vi "Check Status No Objects - Function Generator.vi"(8 "error in (no error)":errorcluster, 10 "VISA Resource Name":refnum<visa-resource-name>="USB0::0x0699::0x0345::C010595::INSTR", 11 "Input Cluster":T3={"Ch2"={"General Settings"={" Frequency"=0.0, " Phase"=0.0, " Run Mode"=0, " Waveform Shape"=0, "Output on?"=FALSE}, "Voltage Settings"={"Amplitude"=0.0, "Offset"=0.0}, "Ramp Settings"={"Ramp Symmetry (%)"=50.0}, "Pulse Settings"={"Leading Edge Time "=5e-09, "Trailing Edge Time"=5e-09, "Duty Cycle (%)"=50.0}, "Sweep Mode Settings"={"Start Freq. "=0.0, "Stop Freq.  "=0.0, "Sweep spacing"=0, "Sweep time"=0.0, "Hold time"=0.0, "Return time"=0.0}, "Burst Mode Settings"={"Burst Mode "=1, "Burst Count"=5}, "AM Settings"={"AM Source "=0, "Modulation Waveform "=0, "Modulation Frequency "=1000.0, "Modulation Depth "=0.0}, "FM Settings"={"FM Source "=0, "Modulation Waveform "=0, "Modulation Frequency"=100.0, "Peak Deviation "=100.0}}, "Ch1"={"General Settings"={" Frequency"=0.0, " Phase"=0.0, " Run Mode"=0, " Waveform Shape"=0, "Output on?"=FALSE}, "Voltage Settings"={"Amplitude"=0.0, "Offset"=0.0}, "Ramp Settings"={"Ramp Symmetry (%)"=50.0}, "Pulse Settings"={"Leading Edge Time "=5e-09, "Trailing Edge Time"=5e-09, "Duty Cycle (%)"=50.0}, "Sweep Mode Settings"={"Start Freq. "=0.0, "Stop Freq.  "=0.0, "Sweep spacing"=0, "Sweep time"=0.0, "Hold time"=0.0, "Return time"=0.0}, "Burst Mode Settings"={"Burst Mode "=1, "Burst Count"=5}, "AM Settings"={"AM Source "=0, "Modulation Waveform "=0, "Modulation Frequency "=1000.0, "Modulation Depth "=0.0}, "FM Settings"={"FM Source "=0, "Modulation Waveform "=0, "Modulation Frequency"=100.0, "Peak Deviation "=100.0}}} {"Ch1"."General Settings"."Waveform Shape" items=["Sinusoid", "Square", "Pulse", "Ramp", "PRNoise", "DC", "SINC", "Gaussian", "Lorentz", "ERise", "EDecay", "Haversine", "User 1", "User 2", "User 3", "User 4", "EMemory", "EFile"]; "Ch1"."General Settings"."Run Mode" items=["Continuous", "AM", "FM", "PM", "FSK", "PWM", "Sweep", "Burst"]; "Ch1"."FM Settings"."Modulation Waveform" items=["Sine", "Square", "Triangle", "Ramp", "Down Ramp", "Noise", "User 1", "User 2", "User 3", "User 4", "EMEMory", "EFILe"]; "Ch1"."FM Settings"."FM Source" items=["Internal", "External"]; "Ch1"."AM Settings"."Modulation Waveform" items=["Sine", "Square", "Triangle", "Ramp", "Down Ramp", "Noise"]; "Ch1"."AM Settings"."AM Source" items=["Internal", "External"]; "Ch1"."Burst Mode Settings"."Burst Mode" items=["Triggered", "Gated"]; "Ch1"."Sweep Mode Settings"."Sweep spacing" items=["linear", "log"]; "Ch1"."Pulse Settings"."Trailing Edge Time" format="%#.6g"; "Ch1"."Pulse Settings"."Leading Edge Time" format="%#.6g"; "Ch1"."Ramp Settings"."Ramp Symmetry (%)" min=0.0 max=100.0 step=1.0 format="%.2f"; "Ch2"."General Settings"."Waveform Shape" items=["Sinusoid", "Square", "Pulse", "Ramp", "PRNoise", "DC", "SINC", "Gaussian", "Lorentz", "ERise", "EDecay", "Haversine", "User 1", "User 2", "User 3", "User 4", "EMemory", "EFile"]; "Ch2"."General Settings"."Run Mode" items=["Continuous", "AM", "FM", "PM", "FSK", "PWM", "Sweep", "Burst"]; "Ch2"."FM Settings"."Modulation Waveform" items=["Sine", "Square", "Triangle", "Ramp", "Down Ramp", "Noise", "User 1", "User 2", "User 3", "User 4", "EMEMory", "EFILe"]; "Ch2"."FM Settings"."FM Source" items=["Internal", "External"]; "Ch2"."AM Settings"."Modulation Waveform" items=["Sine", "Square", "Triangle", "Ramp", "Down Ramp", "Noise"]; "Ch2"."AM Settings"."AM Source" items=["Internal", "External"]; "Ch2"."Burst Mode Settings"."Burst Mode" items=["Triggered", "Gated"]; "Ch2"."Sweep Mode Settings"."Sweep spacing" items=["linear", "log"]; "Ch2"."Pulse Settings"."Trailing Edge Time" format="%#.6g"; "Ch2"."Pulse Settings"."Leading Edge Time" format="%#.6g"; "Ch2"."Ramp Settings"."Ramp Symmetry (%)" min=0.0 max=100.0 step=1.0 format="%.2f"}) -> (0 "error out":errorcluster, 1 "Status":string, 2 "Ready?":bool, 3 "Output Cluster":T3={"Ch2"={"General Settings"={" Frequency"=0.0, " Phase"=0.0, " Run Mode"=0, " Waveform Shape"=0, "Output on?"=FALSE}, "Voltage Settings"={"Amplitude"=0.0, "Offset"=0.0}, "Ramp Settings"={"Ramp Symmetry (%)"=50.0}, "Pulse Settings"={"Leading Edge Time "=5e-09, "Trailing Edge Time"=5e-09, "Duty Cycle (%)"=50.0}, "Sweep Mode Settings"={"Start Freq. "=0.0, "Stop Freq.  "=0.0, "Sweep spacing"=0, "Sweep time"=0.0, "Hold time"=0.0, "Return time"=0.0}, "Burst Mode Settings"={"Burst Mode "=1, "Burst Count"=5}, "AM Settings"={"AM Source "=0, "Modulation Waveform "=0, "Modulation Frequency "=1000.0, "Modulation Depth "=0.0}, "FM Settings"={"FM Source "=0, "Modulation Waveform "=0, "Modulation Frequency"=100.0, "Peak Deviation "=100.0}}, "Ch1"={"General Settings"={" Frequency"=0.0, " Phase"=0.0, " Run Mode"=0, " Waveform Shape"=0, "Output on?"=FALSE}, "Voltage Settings"={"Amplitude"=0.0, "Offset"=0.0}, "Ramp Settings"={"Ramp Symmetry (%)"=50.0}, "Pulse Settings"={"Leading Edge Time "=5e-09, "Trailing Edge Time"=5e-09, "Duty Cycle (%)"=50.0}, "Sweep Mode Settings"={"Start Freq. "=0.0, "Stop Freq.  "=0.0, "Sweep spacing"=0, "Sweep time"=0.0, "Hold time"=0.0, "Return time"=0.0}, "Burst Mode Settings"={"Burst Mode "=1, "Burst Count"=5}, "AM Settings"={"AM Source "=0, "Modulation Waveform "=0, "Modulation Frequency "=1000.0, "Modulation Depth "=0.0}, "FM Settings"={"FM Source "=0, "Modulation Waveform "=0, "Modulation Frequency"=100.0, "Peak Deviation "=100.0}}} {"Ch1"."General Settings"."Waveform Shape" items=["Sinusoid", "Square", "Pulse", "Ramp", "PRNoise", "DC", "SINC", "Gaussian", "Lorentz", "ERise", "EDecay", "Haversine", "User 1", "User 2", "User 3", "User 4", "EMemory", "EFile"]; "Ch1"."General Settings"."Run Mode" items=["Continuous", "AM", "FM", "PM", "FSK", "PWM", "Sweep", "Burst"]; "Ch1"."FM Settings"."Modulation Waveform" items=["Sine", "Square", "Triangle", "Ramp", "Down Ramp", "Noise", "User 1", "User 2", "User 3", "User 4", "EMEMory", "EFILe"]; "Ch1"."FM Settings"."FM Source" items=["Internal", "External"]; "Ch1"."AM Settings"."Modulation Waveform" items=["Sine", "Square", "Triangle", "Ramp", "Down Ramp", "Noise"]; "Ch1"."AM Settings"."AM Source" items=["Internal", "External"]; "Ch1"."Burst Mode Settings"."Burst Mode" items=["Triggered", "Gated"]; "Ch1"."Sweep Mode Settings"."Sweep spacing" items=["linear", "log"]; "Ch1"."Pulse Settings"."Trailing Edge Time" format="%#.6g"; "Ch1"."Pulse Settings"."Leading Edge Time" format="%#.6g"; "Ch1"."Ramp Settings"."Ramp Symmetry (%)" min=0.0 max=100.0 step=1.0 format="%.2f"; "Ch2"."General Settings"."Waveform Shape" items=["Sinusoid", "Square", "Pulse", "Ramp", "PRNoise", "DC", "SINC", "Gaussian", "Lorentz", "ERise", "EDecay", "Haversine", "User 1", "User 2", "User 3", "User 4", "EMemory", "EFile"]; "Ch2"."General Settings"."Run Mode" items=["Continuous", "AM", "FM", "PM", "FSK", "PWM", "Sweep", "Burst"]; "Ch2"."FM Settings"."Modulation Waveform" items=["Sine", "Square", "Triangle", "Ramp", "Down Ramp", "Noise", "User 1", "User 2", "User 3", "User 4", "EMEMory", "EFILe"]; "Ch2"."FM Settings"."FM Source" items=["Internal", "External"]; "Ch2"."AM Settings"."Modulation Waveform" items=["Sine", "Square", "Triangle", "Ramp", "Down Ramp", "Noise"]; "Ch2"."AM Settings"."AM Source" items=["Internal", "External"]; "Ch2"."Burst Mode Settings"."Burst Mode" items=["Triggered", "Gated"]; "Ch2"."Sweep Mode Settings"."Sweep spacing" items=["linear", "log"]; "Ch2"."Pulse Settings"."Trailing Edge Time" format="%#.6g"; "Ch2"."Pulse Settings"."Leading Edge Time" format="%#.6g"; "Ch2"."Ramp Settings"."Ramp Symmetry (%)" min=0.0 max=100.0 step=1.0 format="%.2f"})   [LabVIEW 2012]
doc: "Checks if the instrument is powered on and updates its member data with the instrument's current status."
uses:
  Tektronix AFG 3000 Series/controls.llb/Waveform Shape.ctl
  Tektronix AFG 3000 Series/controls.llb/Sweep Spacing.ctl
  Tektronix AFG 3000 Series/controls.llb/Sweep Time Parameter.ctl
  Tektronix AFG 3000 Series/controls.llb/Sweep Frequency.ctl
  Tektronix AFG 3000 Series/controls.llb/Voltage.ctl
  Tektronix AFG 3000 Series/Tektronix AFG 3000 Series.lvlib
panel:
  in  "Channel Settings":T4={"General Settings"={" Frequency"=0.0, " Phase"=0.0, " Run Mode"=0, " Waveform Shape"=0, "Output on?"=FALSE}, "Voltage Settings"={"Amplitude"=0.0, "Offset"=0.0}, "Ramp Settings"={"Ramp Symmetry (%)"=50.0}, "Pulse Settings"={"Leading Edge Time "=5e-09, "Trailing Edge Time"=5e-09, "Duty Cycle (%)"=50.0}, "Sweep Mode Settings"={"Start Freq. "=0.0, "Stop Freq.  "=0.0, "Sweep spacing"=0, "Sweep time"=0.0, "Hold time"=0.0, "Return time"=0.0}, "Burst Mode Settings"={"Burst Mode "=1, "Burst Count"=5}, "AM Settings"={"AM Source "=0, "Modulation Waveform "=0, "Modulation Frequency "=1000.0, "Modulation Depth "=0.0}, "FM Settings"={"FM Source "=0, "Modulation Waveform "=0, "Modulation Frequency"=100.0, "Peak Deviation "=100.0}} {"General Settings"."Waveform Shape" items=["Sinusoid", "Square", "Pulse", "Ramp", "PRNoise", "DC", "SINC", "Gaussian", "Lorentz", "ERise", "EDecay", "Haversine", "User 1", "User 2", "User 3", "User 4", "EMemory", "EFile"]; "General Settings"."Run Mode" items=["Continuous", "AM", "FM", "PM", "FSK", "PWM", "Sweep", "Burst"]; "FM Settings"."Modulation Waveform" items=["Sine", "Square", "Triangle", "Ramp", "Down Ramp", "Noise", "User 1", "User 2", "User 3", "User 4", "EMEMory", "EFILe"]; "FM Settings"."FM Source" items=["Internal", "External"]; "AM Settings"."Modulation Waveform" items=["Sine", "Square", "Triangle", "Ramp", "Down Ramp", "Noise"]; "AM Settings"."AM Source" items=["Internal", "External"]; "Burst Mode Settings"."Burst Mode" items=["Triggered", "Gated"]; "Sweep Mode Settings"."Sweep spacing" items=["linear", "log"]; "Pulse Settings"."Trailing Edge Time" format="%#.6g"; "Pulse Settings"."Leading Edge Time" format="%#.6g"; "Ramp Settings"."Ramp Symmetry (%)" min=0.0 max=100.0 step=1.0 format="%.2f"}
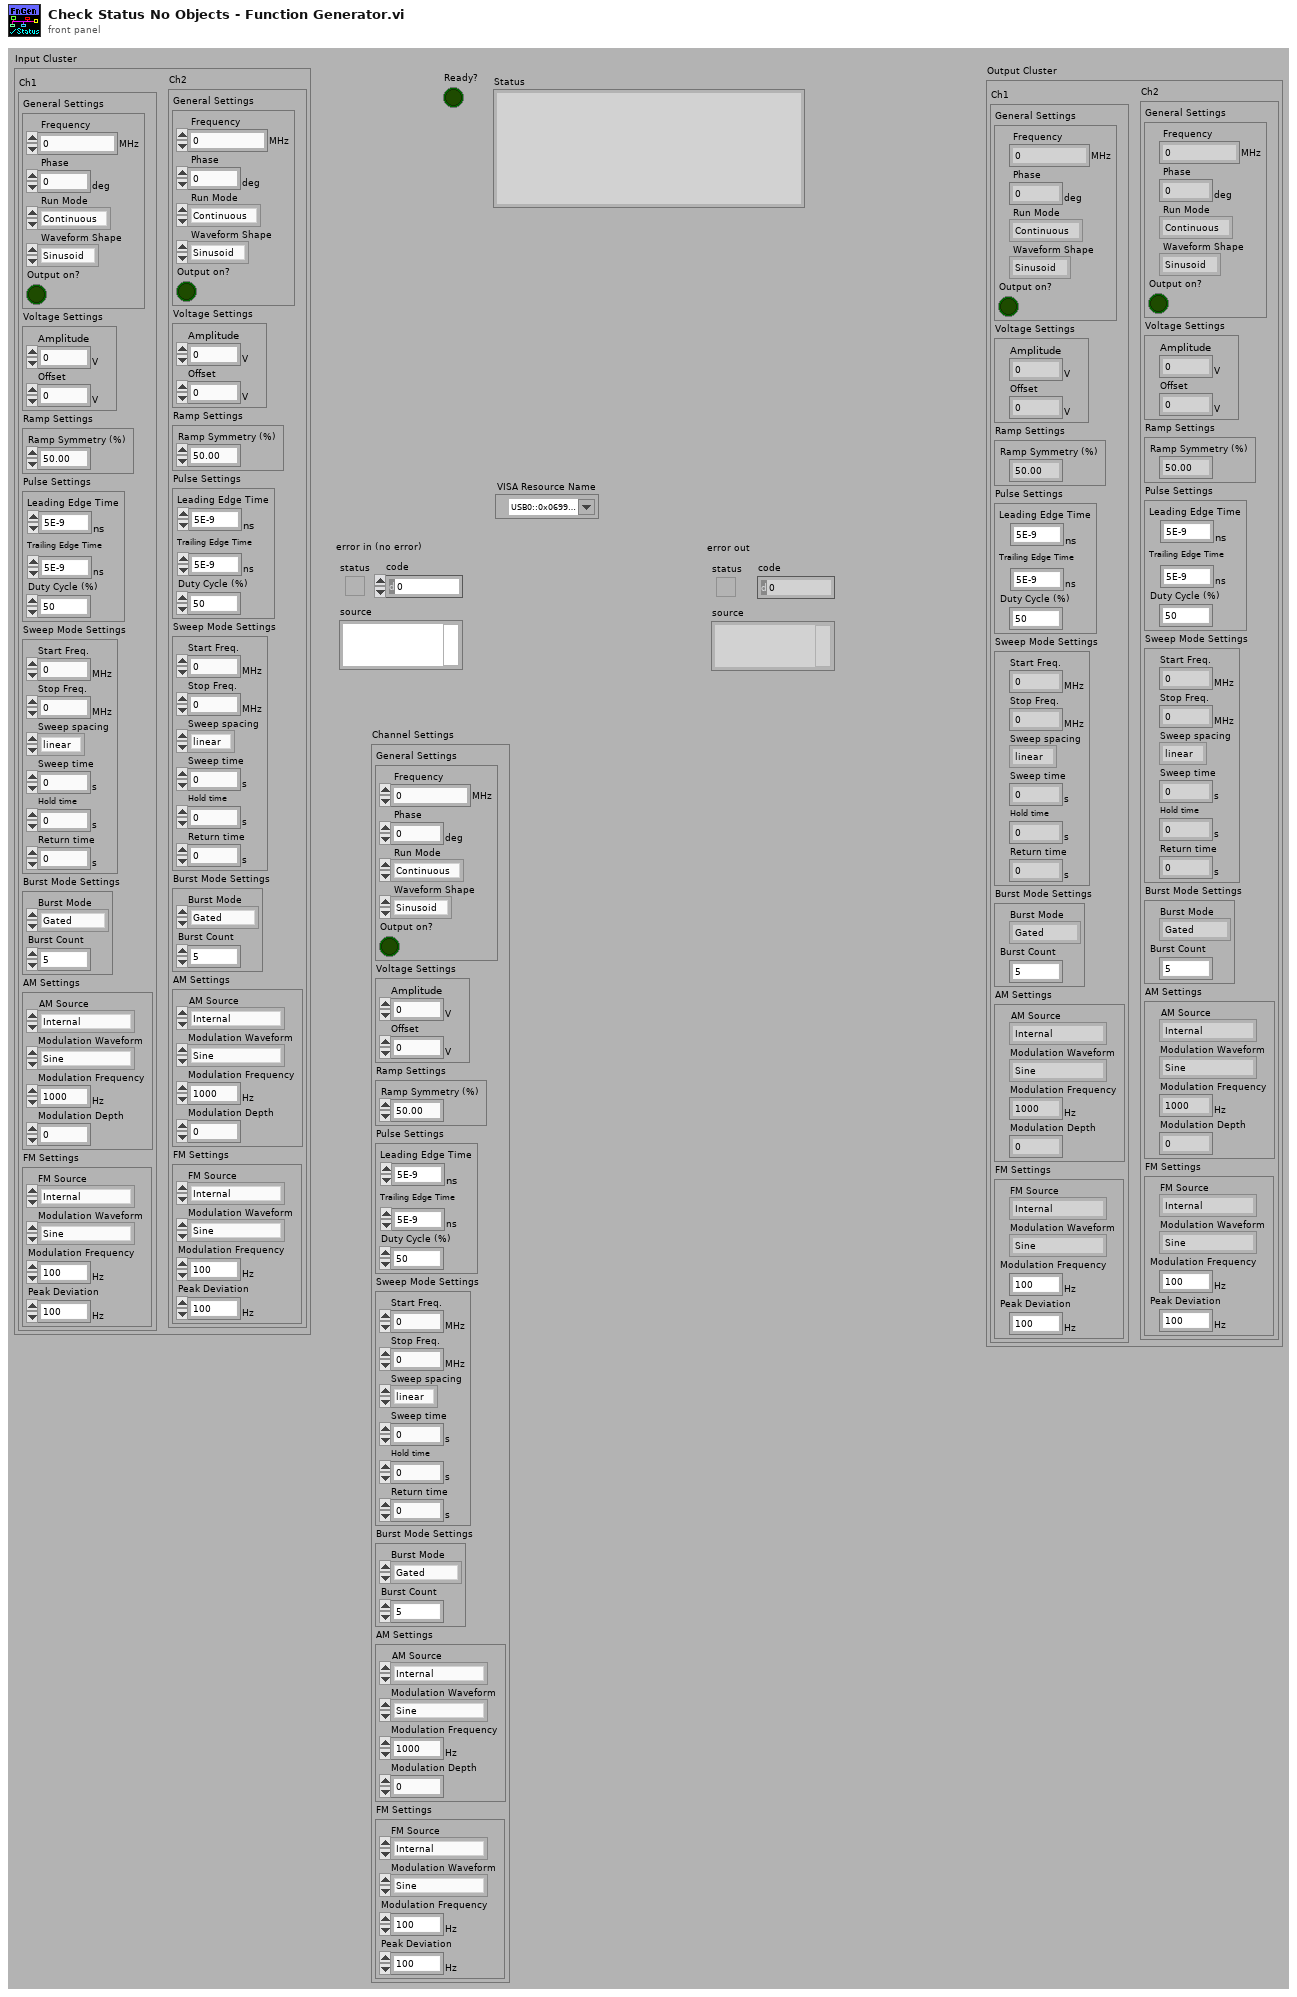
[diagram p1: front panel]
types:
  T1 = typedef "Waveform Shape.ctl" = u16
  T2 = typedef "Sweep Spacing.ctl" = u16
  T3 = cluster{"Ch2":cluster{"General Settings":cluster{" Frequency":dbl[unit], " Phase":dbl[unit], " Run Mode":u16, " Waveform Shape":T1, "Output on?":bool}, "Voltage Settings":cluster{"Amplitude":dbl[unit], "Offset":dbl[unit]}, "Ramp Settings":cluster{"Ramp Symmetry (%)":dbl}, "Pulse Settings":cluster{"Leading Edge Time ":dbl[unit], "Trailing Edge Time":dbl[unit], "Duty Cycle (%)":dbl}, "Sweep Mode Settings":cluster{"Start Freq. ":dbl[unit], "Stop Freq.  ":dbl[unit], "Sweep spacing":T2, "Sweep time":dbl[unit], "Hold time":dbl[unit], "Return time":dbl[unit]}, "Burst Mode Settings":cluster{"Burst Mode ":u16, "Burst Count":i32}, "AM Settings":cluster{"AM Source ":u16, "Modulation Waveform ":u16, "Modulation Frequency ":dbl[unit], "Modulation Depth ":dbl}, "FM Settings":cluster{"FM Source ":u16, "Modulation Waveform ":u16, "Modulation Frequency":dbl[unit], "Peak Deviation ":dbl[unit]}}, "Ch1":cluster{"General Settings":cluster{" Frequency":dbl[unit], " Phase":dbl[unit], " Run Mode":u16, " Waveform Shape":T1, "Output on?":bool}, "Voltage Settings":cluster{"Amplitude":dbl[unit], "Offset":dbl[unit]}, "Ramp Settings":cluster{"Ramp Symmetry (%)":dbl}, "Pulse Settings":cluster{"Leading Edge Time ":dbl[unit], "Trailing Edge Time":dbl[unit], "Duty Cycle (%)":dbl}, "Sweep Mode Settings":cluster{"Start Freq. ":dbl[unit], "Stop Freq.  ":dbl[unit], "Sweep spacing":T2, "Sweep time":dbl[unit], "Hold time":dbl[unit], "Return time":dbl[unit]}, "Burst Mode Settings":cluster{"Burst Mode ":u16, "Burst Count":i32}, "AM Settings":cluster{"AM Source ":u16, "Modulation Waveform ":u16, "Modulation Frequency ":dbl[unit], "Modulation Depth ":dbl}, "FM Settings":cluster{"FM Source ":u16, "Modulation Waveform ":u16, "Modulation Frequency":dbl[unit], "Peak Deviation ":dbl[unit]}}}
  T4 = cluster{"General Settings":cluster{" Frequency":dbl[unit], " Phase":dbl[unit], " Run Mode":u16, " Waveform Shape":T1, "Output on?":bool}, "Voltage Settings":cluster{"Amplitude":dbl[unit], "Offset":dbl[unit]}, "Ramp Settings":cluster{"Ramp Symmetry (%)":dbl}, "Pulse Settings":cluster{"Leading Edge Time ":dbl[unit], "Trailing Edge Time":dbl[unit], "Duty Cycle (%)":dbl}, "Sweep Mode Settings":cluster{"Start Freq. ":dbl[unit], "Stop Freq.  ":dbl[unit], "Sweep spacing":T2, "Sweep time":dbl[unit], "Hold time":dbl[unit], "Return time":dbl[unit]}, "Burst Mode Settings":cluster{"Burst Mode ":u16, "Burst Count":i32}, "AM Settings":cluster{"AM Source ":u16, "Modulation Waveform ":u16, "Modulation Frequency ":dbl[unit], "Modulation Depth ":dbl}, "FM Settings":cluster{"FM Source ":u16, "Modulation Waveform ":u16, "Modulation Frequency":dbl[unit], "Peak Deviation ":dbl[unit]}}
  T5 = typedef "Voltage.ctl" = enum16{"amplitude", "offset", "high", "low", "high limit", "low limit"}
  T6 = typedef "Sweep Frequency.ctl" = enum16{"center", "span", "start", "stop"}
  T7 = typedef "Sweep Time Parameter.ctl" = enum16{"sweep time", "hold time", "return time"}
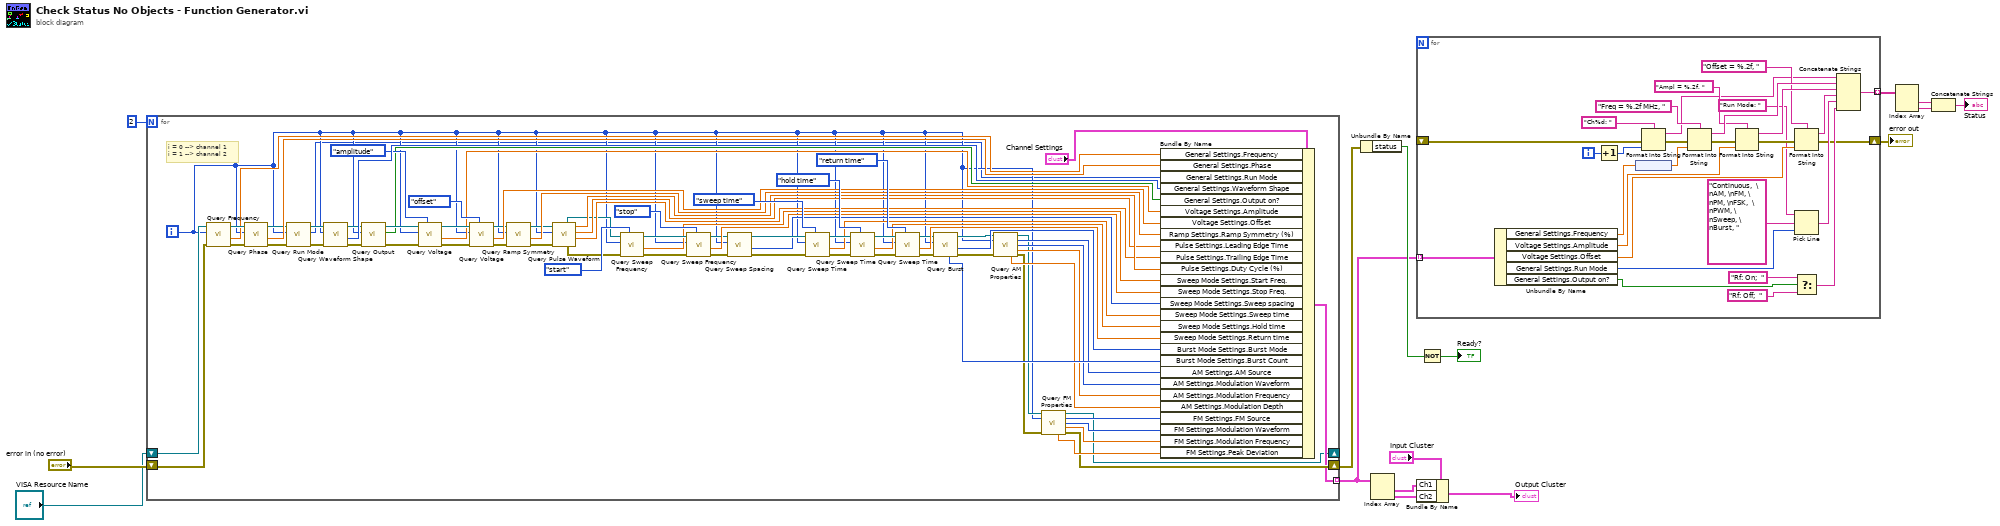
[diagram p0: block diagram]
diagram:
  n1 = for {
    N: 2 -> [_]
    shift-right: [w33] -> w14
    shift-left: "error in (no error)" -> [w82]
    tunnel: [w32] -> w13 mode=indexing
    shift-right: [w31] -> _
    shift-left: "VISA Resource Name" -> [w30]
    i -> [w19]
    # "i = 0 --> channel 1\ni = 1 --> channel 2"
    n2 = call "Query Frequency.vi"("error in (no error)"=w82, "Channel (0: Channel 1)"=w19, "VISA resource name"=w30) -> ("error out"=w81:errorcluster, "frequency"=w80:dbl[unit], "VISA resource name out"=w88:refnum<visa-resource-name>)  [unwired: 6 out]
    n3 = call "Query Phase.vi"("error in (no error)"=w81, "Channel (0: Channel 1)"=w19, "VISA resource name"=w88) -> ("error out"=w21:errorcluster, "phase"=w79:dbl[unit], "VISA resource name out"=w23:refnum<visa-resource-name>)  [unwired: 6 out]
    n4 = call "Query Run Mode.vi"("error in (no error)"=w21, "Channel (0: Channel 1)"=w19, "VISA resource name"=w23) -> ("error out"=w20:errorcluster, "Run Mode"=w18:u16, "VISA resource name out"=w22:refnum<visa-resource-name>)  [unwired: 6 out]
    n5 = call "Query Waveform Shape.vi"("error in (no error)"=w20, "Channel (0: Channel 1)"=w19, "VISA resource name"=w22) -> ("error out"=w26:errorcluster, "Waveform Shape"=w78:T1, "VISA resource name out"=w28:refnum<visa-resource-name>)  [unwired: 6 out]
    n6 = call "Query Output.vi"("error in (no error)"=w26, "Channel (0: Channel 1)"=w19, "VISA resource name"=w28) -> ("error out"=w25:errorcluster, "Output Enabled?"=w24:bool, "VISA resource name out"=w27:refnum<visa-resource-name>)  [unwired: 6 out]
    n7 = call "Query Voltage.vi"("Voltage Param (amplitude)"=Voltage."amplitude", "error in (no error)"=w25, "Channel (0: Channel 1)"=w19, "VISA resource name"=w27) -> ("error out"=w45:errorcluster, "voltage"=w29:dbl[unit], "VISA resource name out"=w75:refnum<visa-resource-name>)  [unwired: 5 out]
    n8 = call "Query Voltage.vi"("Voltage Param (amplitude)"=Voltage."offset", "error in (no error)"=w45, "Channel (0: Channel 1)"=w19, "VISA resource name"=w75) -> ("error out"=w44:errorcluster, "voltage"=w74:dbl[unit], "VISA resource name out"=w73:refnum<visa-resource-name>)  [unwired: 5 out]
    n9 = call "Query Ramp Symmetry.vi"("error in (no error)"=w44, "Channel (0: Channel 1)"=w19, "VISA resource name"=w73) -> ("error out"=w43:errorcluster, "Symmetry (%)"=w72:dbl, "VISA resource name out"=w71:refnum<visa-resource-name>)  [unwired: 6 out]
    n10 = call "Query Pulse Waveform.vi"("error in (no error)"=w43, "Channel (0: Channel 1)"=w19, "VISA resource name"=w71) -> ("Trailing"=w68:dbl[unit], "Leading"=w69:dbl[unit], "Duty Cycle"=w70:dbl, "error out"=w42:errorcluster, "VISA resource name out"=w67:refnum<visa-resource-name>)  [unwired: 4 out]
    n11 = call "Query Sweep Frequency.vi"("Sweep Frequency"=Sweep_Frequency."start", "error in (no error)"=w42, "Channel (0: Channel 1)"=w19, "VISA resource name"=w67) -> ("error out"=w41:errorcluster, "frequency"=w66:dbl[unit], "VISA resource name out"=w91:refnum<visa-resource-name>)  [unwired: 5 out]
    n12 = call "Query Sweep Frequency.vi"("Sweep Frequency"=Sweep_Frequency."stop", "error in (no error)"=w41, "Channel (0: Channel 1)"=w19, "VISA resource name"=w91) -> ("error out"=w40:errorcluster, "frequency"=w65:dbl[unit], "VISA resource name out"=w64:refnum<visa-resource-name>)  [unwired: 5 out]
    n13 = call "Query Sweep Spacing.vi"("error in (no error)"=w40, "Channel (0: Channel 1)"=w19, "VISA resource name"=w64) -> ("error out"=w39:errorcluster, "Sweep spacing (linear)"=w62:T2, "VISA resource name out"=w63:refnum<visa-resource-name>)  [unwired: 6 out]
    n14 = call "Query Sweep Time.vi"("Sweep Time Param (sweep time)"=Sweep_Time_Parameter."sweep time", "error in (no error)"=w39, "Channel (0: Channel 1)"=w19, "VISA resource name"=w63) -> ("error out"=w38:errorcluster, "time"=w61:dbl[unit], "VISA resource name out"=w89:refnum<visa-resource-name>)  [unwired: 5 out]
    n15 = call "Query Sweep Time.vi"("Sweep Time Param (sweep time)"=Sweep_Time_Parameter."hold time", "error in (no error)"=w38, "Channel (0: Channel 1)"=w19, "VISA resource name"=w89) -> ("error out"=w37:errorcluster, "time"=w60:dbl[unit], "VISA resource name out"=w90:refnum<visa-resource-name>)  [unwired: 5 out]
    n16 = call "Query Sweep Time.vi"("Sweep Time Param (sweep time)"=Sweep_Time_Parameter."return time", "error in (no error)"=w37, "Channel (0: Channel 1)"=w19, "VISA resource name"=w90) -> ("error out"=w36:errorcluster, "time"=w59:dbl[unit], "VISA resource name out"=w58:refnum<visa-resource-name>)  [unwired: 5 out]
    n17 = call "Query Burst.vi"("error in (no error)"=w36, "Channel (0: Channel 1)"=w19, "VISA resource name"=w58) -> ("error out"=w35:errorcluster, "Burst Mode"=w57:u16, "VISA resource name out"=w55:refnum<visa-resource-name>, "Burst Count"=w56:i32)  [unwired: 5 out]
    n18 = call "Query AM Properties.vi"("VISA resource name"=w55, "Channel (0: Channel 1)"=w19, "error in (no error)"=w35) -> ("VISA resource name out"=w50:refnum<visa-resource-name>, "AM Source"=w54:u16, "Modulation Waveform"=w53:u16, "Modulation Frequency"=w52:dbl[unit], "Modulation Depth"=w51:dbl, "error out"=w34:errorcluster)  [unwired: 7 out]
    n19 = call "Query FM Properties.vi"("VISA resource name"=w50, "Channel (0: Channel 1)"=w19, "error in (no error)"=w34) -> ("VISA resource name out"=w31:refnum<visa-resource-name>, "FM Source"=w49:u16, "Modulation Waveform"=w48:u16, "Modulation Frequency"=w47:dbl[unit], "Peak Deviation"=w46:dbl[unit], "error out"=w33:errorcluster)  [unwired: 7 out]
    n20 = Bundle By Name(cluster="Channel Settings", "General Settings.Frequency"=w80, "General Settings.Phase"=w79, "General Settings.Run Mode"=w18, "General Settings.Waveform Shape"=w78, "General Settings.Output on?"=w24, "Voltage Settings.Amplitude"=w29, "Voltage Settings.Offset"=w74, "Ramp Settings.Ramp Symmetry (%)"=w72, "Pulse Settings.Leading Edge Time"=w69, "Pulse Settings.Trailing Edge Time"=w68, "Pulse Settings.Duty Cycle (%)"=w70, "Sweep Mode Settings.Start Freq."=w66, "Sweep Mode Settings.Stop Freq."=w65, "Sweep Mode Settings.Sweep spacing"=w62, "Sweep Mode Settings.Sweep time"=w61, "Sweep Mode Settings.Hold time"=w60, "Sweep Mode Settings.Return time"=w59, "Burst Mode Settings.Burst Mode"=w57, "Burst Mode Settings.Burst Count"=w56, "AM Settings.AM Source"=w54, "AM Settings.Modulation Waveform"=w53, "AM Settings.Modulation Frequency"=w52, "AM Settings.Modulation Depth"=w51, "FM Settings.FM Source"=w49, "FM Settings.Modulation Waveform"=w48, "FM Settings.Modulation Frequency"=w47, "FM Settings.Peak Deviation"=w46) -> (w32:T4)
  }
  n21 = Unbundle By Name(w14) -> ("status"=w16:bool)
  n22 = Index Array(array=w13) -> (element #1=w4:T4, element #2=w5:T4)  [unwired: 2 in]
  n23 = for {
    tunnel: w13 -> [w103] mode=indexing
    shift-right: [w97] -> w12
    shift-left: _ -> [w96]
    tunnel: [w95] -> w11 mode=indexing
    i -> [w102]
    n24 = Unbundle By Name(w103) -> ("General Settings.Frequency"=w120:dbl[unit], "Voltage Settings.Amplitude"=w118:dbl[unit], "Voltage Settings.Offset"=w117:dbl[unit], "General Settings.Run Mode"=w116:u16, "General Settings.Output on?"=w115:bool)
    n25 = Increment(x=w102) -> (x+1=w92:i32)
    n26 = node(w120) -> (w119:dbl)
    n27 = Format Into String(format string="Ch%d: " ("string (\"\")"), error in=w96, w92) -> (resulting string=w94:string, error out=w100:errorcluster)  [unwired: 1 in]
    n28 = Format Into String(format string="Freq = %.2f MHz, " ("string (\"\")"), error in=w100, w119) -> (resulting string=w111:string, error out=w99:errorcluster)  [unwired: 1 in]
    n29 = Format Into String(format string="Ampl = %.2f, " ("string (\"\")"), error in=w99, w118) -> (resulting string=w108:string, error out=w98:errorcluster)  [unwired: 1 in]
    n30 = Format Into String(format string="Offset = %.2f, " ("string (\"\")"), error in=w98, w117) -> (resulting string=w106:string, error out=w97:errorcluster)  [unwired: 1 in]
    n31 = Pick Line(string ("")="Run Mode: ", multi-line string="Continuous,  \nAM, \nFM, \nPM, \nFSK,  \nPWM, \nSweep, \nBurst, ", line index=w116) -> (output string=w104:string)
    n32 = Select(t="Rf: On;  " ("string (\"\")"), s=w115, f="Rf: Off;  " ("string (\"\")")) -> (s? t:f=w105:string)
    n33 = Concatenate Strings(w94, w111, w108, w106, w104, w105) -> (w95:string)
  }
  "error out" <- w12
  n34 = Bundle By Name(cluster="Input Cluster", "Ch1"=w4, "Ch2"=w5) -> (→"Output Cluster":T3)
  n35 = Not(x=w16) -> (.not. x?=→"Ready?":bool)
  n36 = Index Array(array=w11) -> (element #1=w10:string, element #2=w9:string)  [unwired: 2 in]
  n37 = Concatenate Strings(w10, w9) -> (→"Status":string)
